vi "Utility - Open-Close Panes.vi"(7 "Panel Type":enum16{"Open", "Close"}(ring), 8 "error in (no error)":errorcluster, 10 "VI Reference In":refnum<vi>, 11 "FilePath":path) -> (0 "error out":errorcluster, 3 "VI Reference Out":refnum<vi>)   [LabVIEW 2014]
panel:
  in  "Front Panel Window:Open":bool
  # "INPUTS"
  # "OUTPUTS"
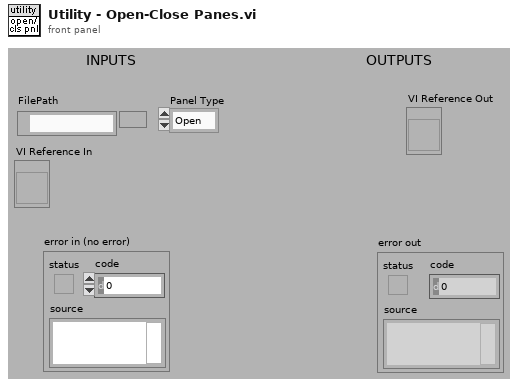
[diagram p1: front panel]
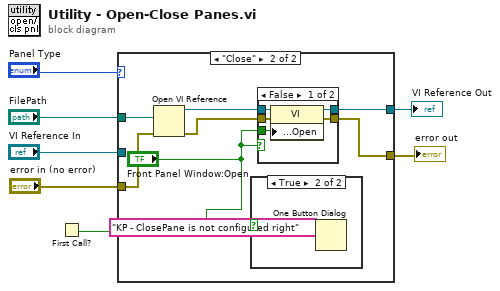
[diagram p0: block diagram]
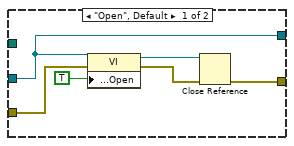
[diagram p2: hidden frame]
diagram:
  n1 = First Call?() -> (First Call?: T/F=w1:bool)
  n2 = case shown="\"Close\"" "Panel Type" {
    tunnel: "FilePath" -> [_ w22]
    tunnel: [w12 w20] -> w6
    tunnel: "VI Reference In" -> [w12 _]
    tunnel: "error in (no error)" -> [w10 w19]
    tunnel: [w8 w17] -> w2
    tunnel: w1 -> [_ w16]
    frame "Open", Default {
      n3 = property class="VI"(reference=w12, error in=w10, "Front Panel Window:Open"=TRUE) -> (reference out=w11:refnum<vi>, error out=w9:errorcluster)
      n4 = Close Reference(reference=w11, error in (no error)=w9) -> (error out=w8:errorcluster)
    }
    frame "Close" {
      n5 = Open VI Reference(vi path=w22, error in (no error)=w19) -> (vi reference=w21:refnum<vi>, error out=w18:errorcluster)  [unwired: 4 out]
      n6 = And(x="Front Panel Window:Open", y=w16) -> (x .and. y?=w15:bool)
      n7 = case shown="True" w15 {
        frame False {
        }
        frame True {
          n8 = One Button Dialog(message="KP - ClosePane is not configured right") -> ()  [unwired: 2 out]
        }
      }
      n9 = case shown="False" "Front Panel Window:Open" {
        tunnel: w21 -> [w27 w29]
        tunnel: [w26 w29] -> w20
        tunnel: w18 -> [w25 w28]
        tunnel: [w24 w28] -> w17
        tunnel: "Front Panel Window:Open" -> [w23 _]
        frame False {
          n10 = property class="VI"(reference=w27, error in=w25, "Front Panel Window:Open"=w23) -> (reference out=w26:refnum<vi>, error out=w24:errorcluster)
        }
        frame True {
        }
      }
    }
  }
  "VI Reference Out" <- w6
  "error out" <- w2
